vi "RFH-utility-common_selector.vi"(9 "size(s)":i32, 10 "XY graph refs":refnum<vi>[](array[refnum])) -> ()   [LabVIEW 2020, in "RFH-Reflection_File_Handler.lvlib"]
uses:
  RFH-Reflection_File_Handler.lvlib
panel:
  out "Numeric":i32
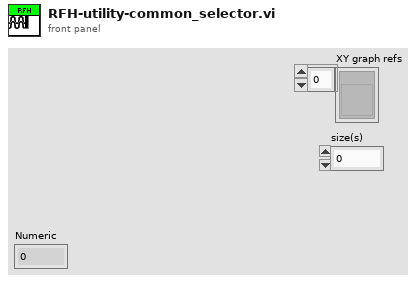
[diagram p1: front panel]
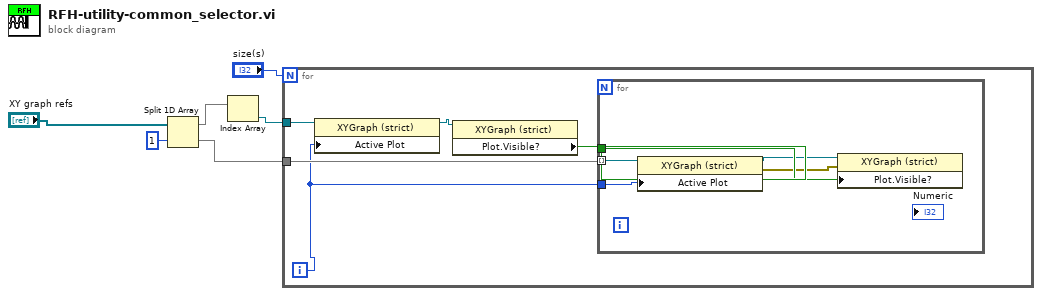
[diagram p0: block diagram]
diagram:
  n1 = Split 1D Array(array="XY graph refs", index=1) -> (first subarray=w5:refnum<vi>[], second subarray=w4:refnum<vi>[])
  n2 = Index Array(array=w5) -> (element=w3:refnum<vi>)  [unwired: 1 in]
  n3 = for {
    N: "size(s)" -> [_]
    tunnel: w4 -> [w11]
    tunnel: w3 -> [w9]
    i -> [w7]
    n4 = property on="Property Node" class="XYGraph (strict)"(reference=w9, "Active Plot"=w7) -> (reference out=w8:refnum<vi>)  [unwired: 1 in, 1 out]
    n5 = property on="Property Node" class="XYGraph (strict)"(reference=w8) -> ("Plot.Visible?"=w10:bool)  [unwired: 1 in, 2 out]
    n6 = for {
      tunnel: w10 -> [w16]
      tunnel: w11 -> [w15] mode=indexing
      tunnel: w7 -> [w12]
      n7 = property on="Property Node" class="XYGraph (strict)"(reference=w15, "Active Plot"=w12) -> (reference out=w14:refnum<vi>, error out=w13:errorcluster)  [unwired: 1 in]
      n8 = property on="Property Node" class="XYGraph (strict)"(reference=w14, error in=w13, "Plot.Visible?"=w16) -> ()  [unwired: 2 out]
    }
  }
